vi "BRig_Host_panel_AnalogInput_v0,40.vi"(9 "graph_ai1":dbl(graph), 10 "graph_ai0":dbl(graph)) -> ()   [LabVIEW 2014]
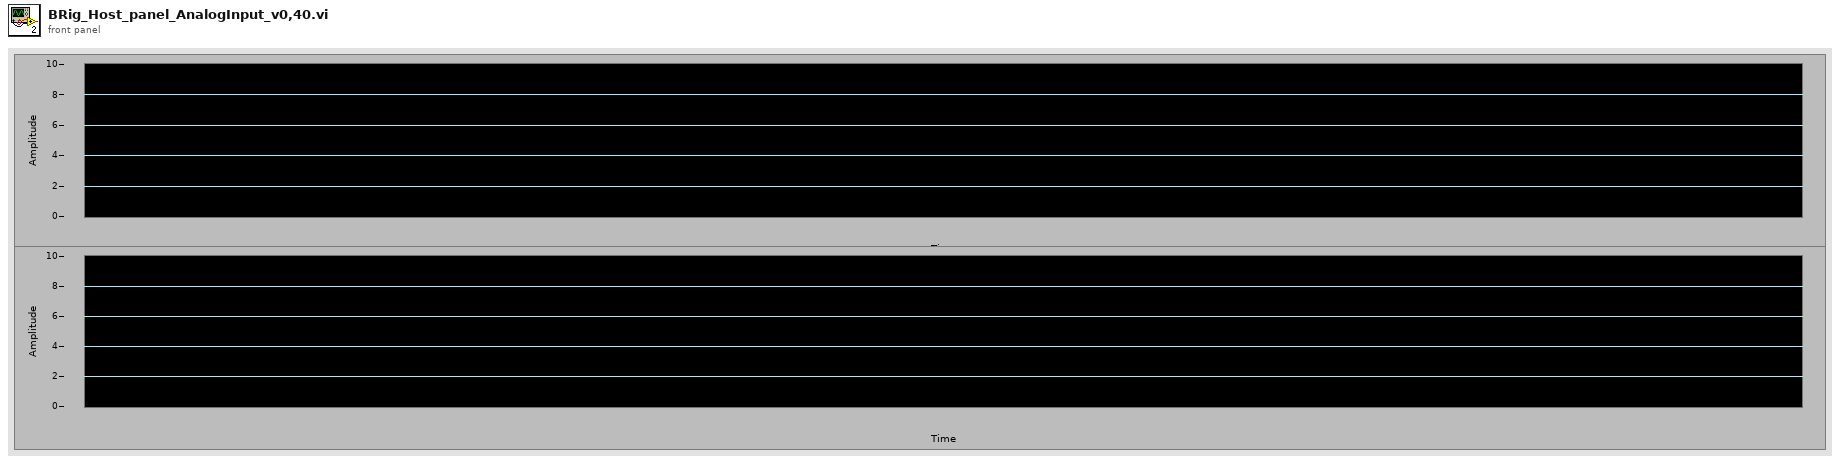
[diagram p1: front panel]
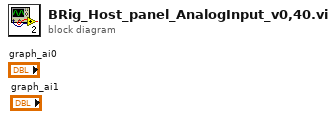
[diagram p0: block diagram]
diagram:
